vi "VisualizeModules.vi"() -> ()   [LabVIEW 2016]
uses:
  2_ModulePositioning/SingleModuleProgressReport.ctl
  <vilib>/vision/driver/NI_Vision_Acquisition_Software.lvlib
  <vilib>/vision/NI_Vision_Development_Module.lvlib
panel:
  in  "Calibration [um/pix]":dbl=0.25
  out "delta Y":sgl
  out "delta X":sgl
  out "Current Position":T1
  in  "Axis Speeds":T2={"X [mm/s]"=25.0, "Y [mm/s]"=12.5, "Z [mm/s]"=5.0}
  in  "stop":bool
  out "Placement Monitor":T3(plugin-control)
  out "appended path":path
  out "Fiducial Template":T3(plugin-control)
  in  "Templates path":path=path "C:/Users/Aerotech/Documents/BNL_ThermomechanicalStave/0_Calibration"
  in  "Module fiducial marker":T4(ring)=enum."[None]"
  out "Module Progress Report":T5(array[cluster])
  in  "Camera Name":refnum<k21>="cam0" caption="IMAQdx Session"
  in  "N modules":i32
  in  "Calibrated positions of fiducials [mm]":dbl[][](array[numeric])=[[-675.4228165149058, -196.82430550413875, -11.55], [-579.8428201474238, -196.8506568257386, -11.55], [-579.816468825824, -101.27066045825673, -11.55], [-675.3964651933059, -101.24430913665685, -11.55], [-577.422820239396, -196.8513240176017, -11.55], [-481.84282387191405, -196.87767533920157, -11.55], [-481.8164725503142, -101.29767897171968, -11.55], [-577.396468917796, -101.2713276501198, -11.55], [-479.42282396388623, -196.87834253106465, -11.55], [-383.8428275964043, -196.90469385266454, -11.55], [-383.81647627480436, -101.32469748518264, -11.55], [-479.3964726422863, -101.29834616358275, -11.55], [-381.42282768837646, -196.90536104452758, -11.55], [-285.8428313208945, -196.93171236612747, -11.55], [-285.8164799992946, -101.35171599864559, -11.55], [-381.39647636677654, -101.3253646770457, -11.55], [-283.4228314128667, -196.93237955799054, -11.55], [-187.84283504538473, -196.95873087959043, -11.55], [-187.8164837237848, -101.37873451210854, -11.55], [-283.39648009126677, -101.35238319050865, -11.55], [-185.42283513735697, -196.9593980714535, -11.55], [-89.84283876987502, -196.98574939305337, -11.55], [-89.81648744827521, -101.40575302557149, -11.55], [-185.39648381575705, -101.3794017039716, -11.55], [-87.42283886184703, -196.98641658491644, -11.55], [8.157157505634814, -197.01276790651633, -11.55], [8.183508827234618, -101.43277153903443, -11.55], [-87.39648754024722, -101.40642021743454, -11.55], [10.57715741366269, -197.01343509837938, -11.55], [106.15715378114453, -197.0397864199793, -11.55], [106.18350510274433, -101.45979005249738, -11.55], [10.603508735262494, -101.4334387308975, -11.55], [108.57715368917252, -197.04045361184234, -11.55], [204.15715005665436, -197.06680493344223, -11.55], [204.18350137825416, -101.48680856596033, -11.55], [108.60350501077232, -101.46045724436046, -11.55], [206.57714996468223, -197.0674721253053, -11.55], [302.1571463321641, -197.09382344690516, -11.55], [302.1834976537639, -101.5138270794233, -11.55], [206.60350128628204, -101.4874757578234, -11.55], [304.57714624019206, -197.09449063876826, -11.55], [400.1571426076739, -197.12084196036813, -11.55], [400.1834939292737, -101.54084559288623, -11.55], [304.60349756179187, -101.51449427128635, -11.55], [402.5771425157018, -197.1215091522312, -11.55], [498.15713888318373, -197.1478604738311, -11.55], [498.18349020478354, -101.56786410634919, -11.55], [402.6034938373016, -101.5415127847493, -11.55], [500.5771387912116, -197.14852766569413, -11.55], [596.1571351586933, -197.17487898729405, -11.55], [596.1834864802931, -101.59488261981214, -11.55], [500.6034901128114, -101.56853129821225, -11.55]]
  # "-101.244"
  # "-196.851"
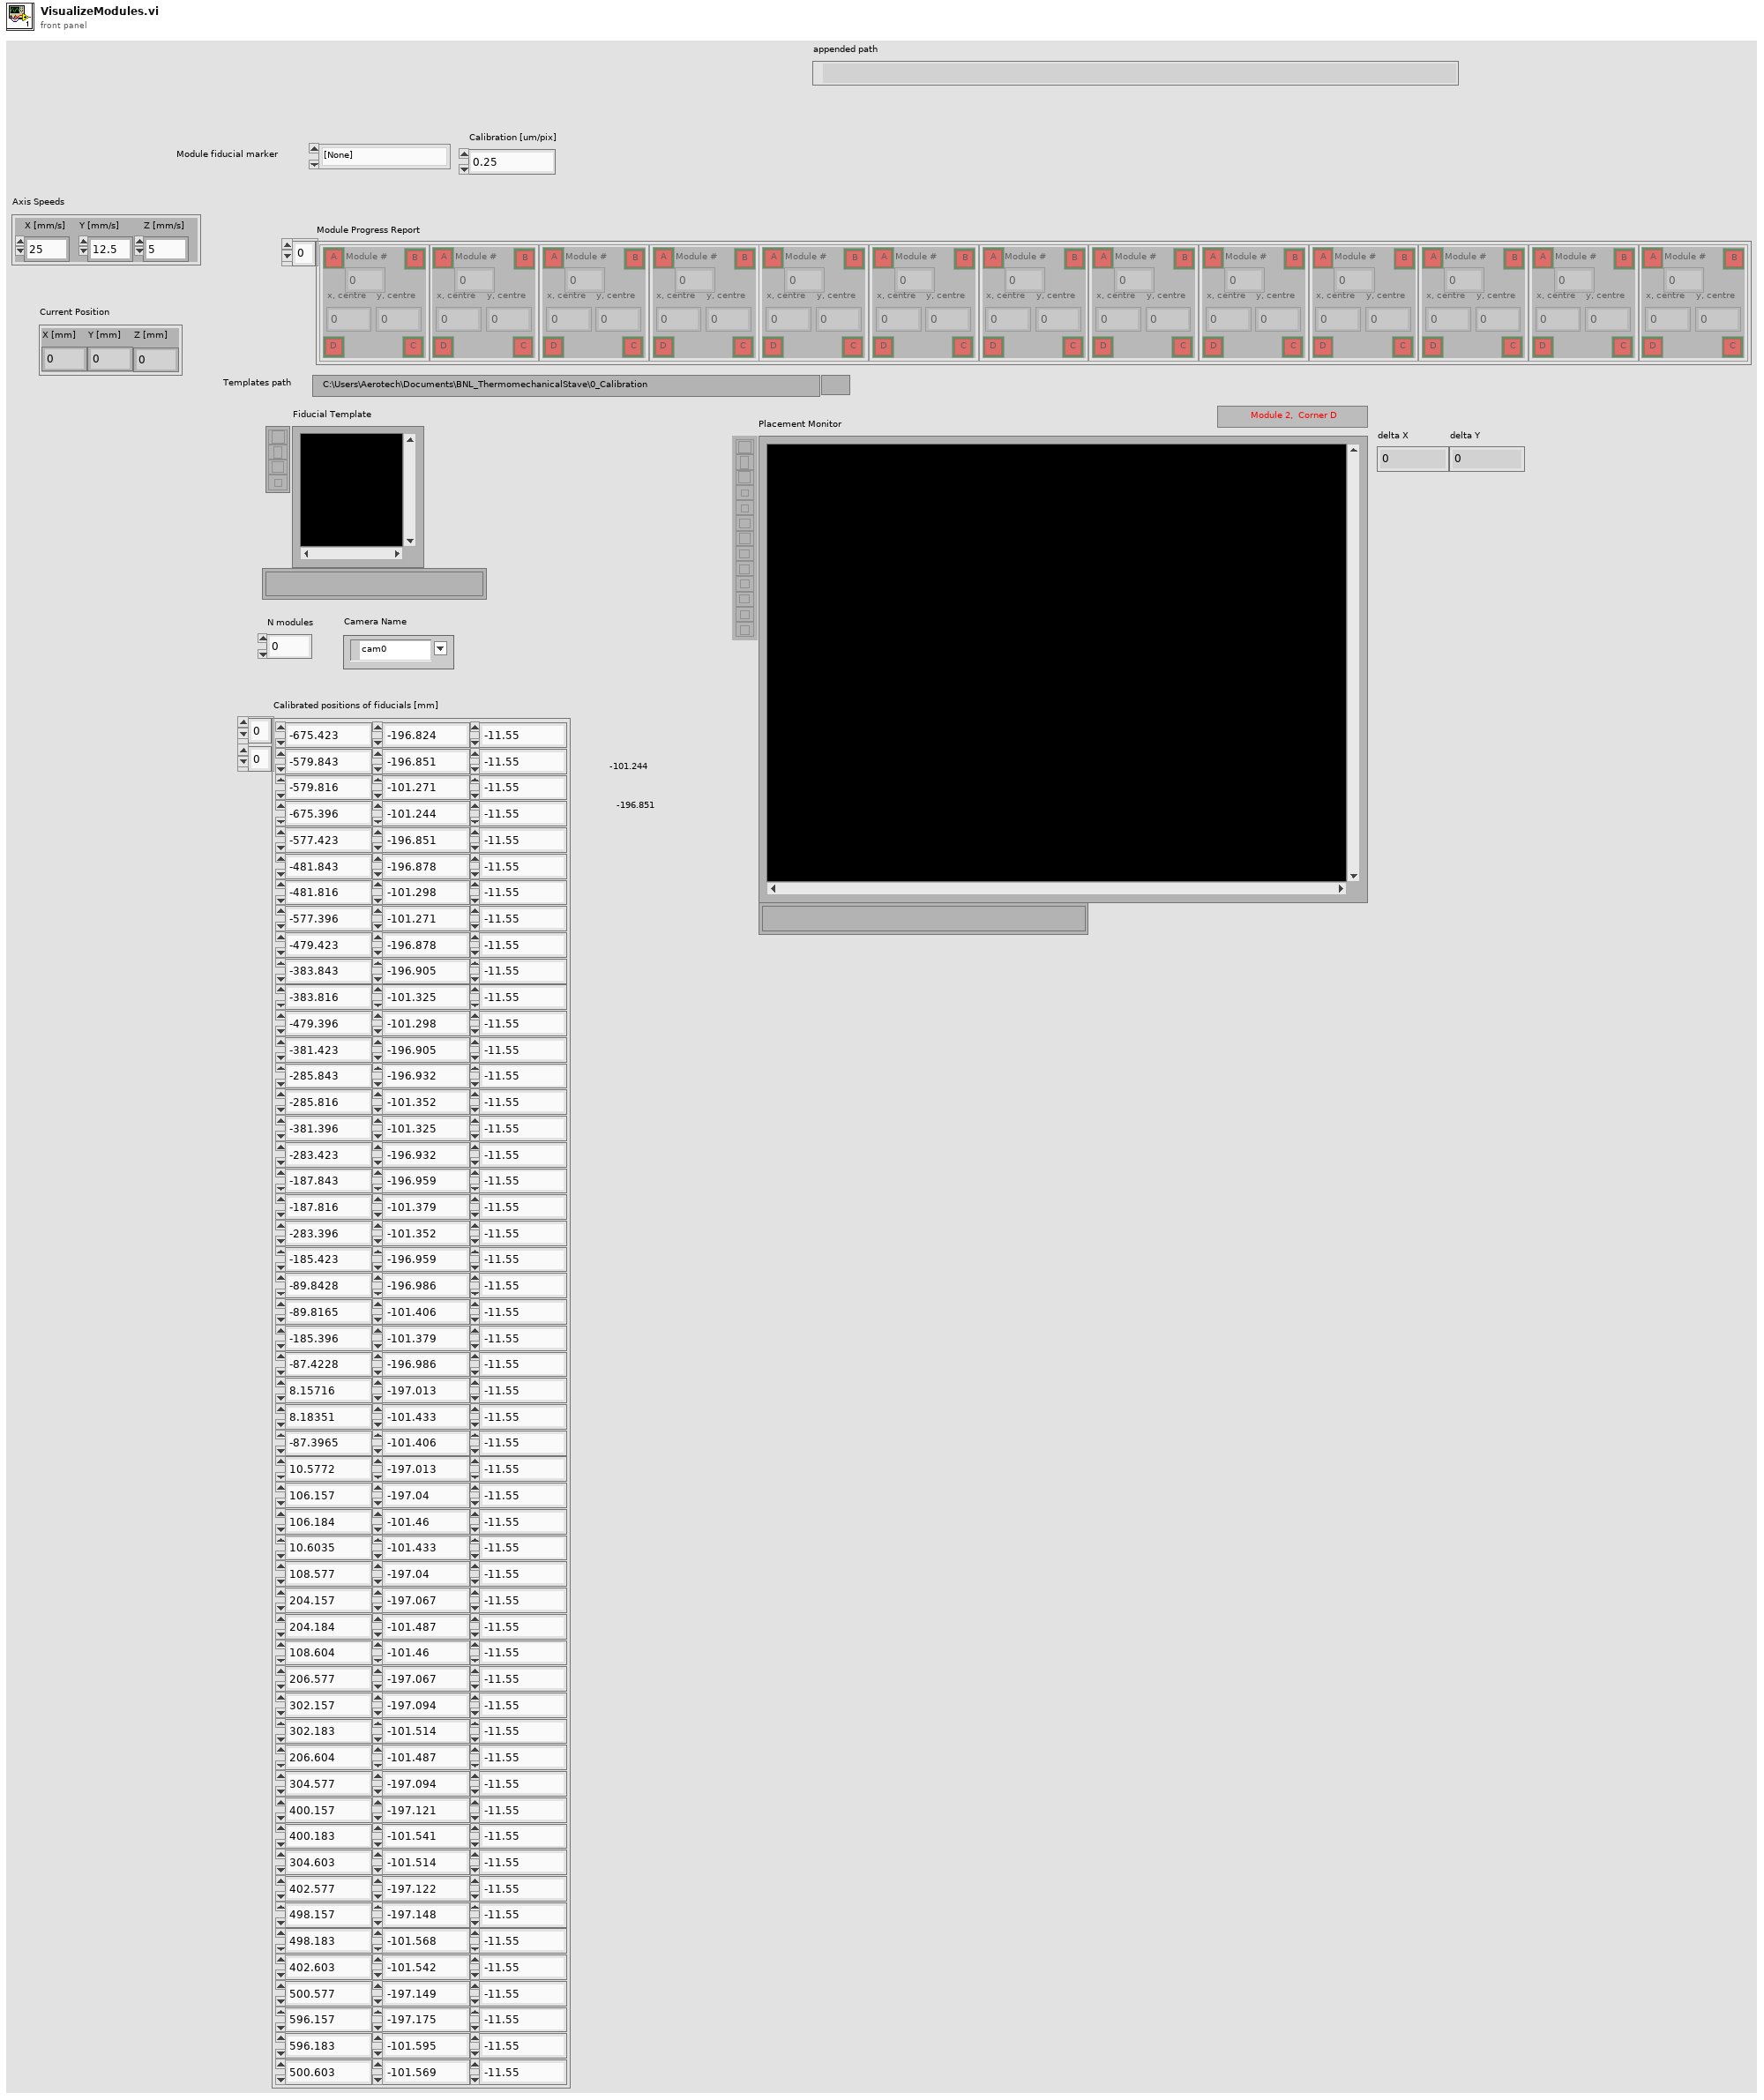
[diagram p1: front panel]
types:
  T1 = cluster{"X [mm]":dbl, "Y [mm]":dbl, "Z [mm]":dbl}
  T2 = cluster{"X [mm/s]":dbl, "Y [mm/s]":dbl, "Z [mm/s]":dbl}
  T3 = typedef "IMAQ Image.ctl" = refnum<image>
  T4 = enum16{"Mark C", "Mark B", "Strip Corner", "[None]"}
  T5 = cluster{"A":bool, "x, centre":dbl, "y, centre":dbl, "Module #":i32, "B":bool, "D":bool, "C":bool}[]
  T6 = typedef "SingleModuleProgressReport.ctl" = cluster{"A":bool, "x, centre":dbl, "y, centre":dbl, "Module #":i32, "B":bool, "D":bool, "C":bool}
  T7 = cluster{"Algorithm":i32, "Number of Matches Requested":i32, "Minimum Match Score":sgl, "SubPixel Accuracy":bool, "Rotation Angle Ranges":cluster{"Start":sgl, "End":sgl}[], "Show Search Area":bool, "Show Result":bool}
  T8 = typedef "IMAQdx.ctl" = refnum<k21>
  T9 = cluster{"Final X":dbl, "Final Y":dbl, "Final Z":dbl}
  T10 = cluster{"Position":cluster{"x":sgl, "y":sgl}, "Angle":sgl, "Scale":sgl, "Score":sgl, "Bounding Box":cluster{"x":sgl, "y":sgl}[]}[]
  T11 = cluster{"Position":cluster{"x":sgl, "y":sgl}, "Angle":sgl, "Scale":sgl, "Score":sgl, "Bounding Box":cluster{"x":sgl, "y":sgl}[]}
  T12 = cluster{"A":bool, "x, centre":dbl, "y, centre":dbl, "Module #":i32, "B":bool, "D":bool, "C":bool}
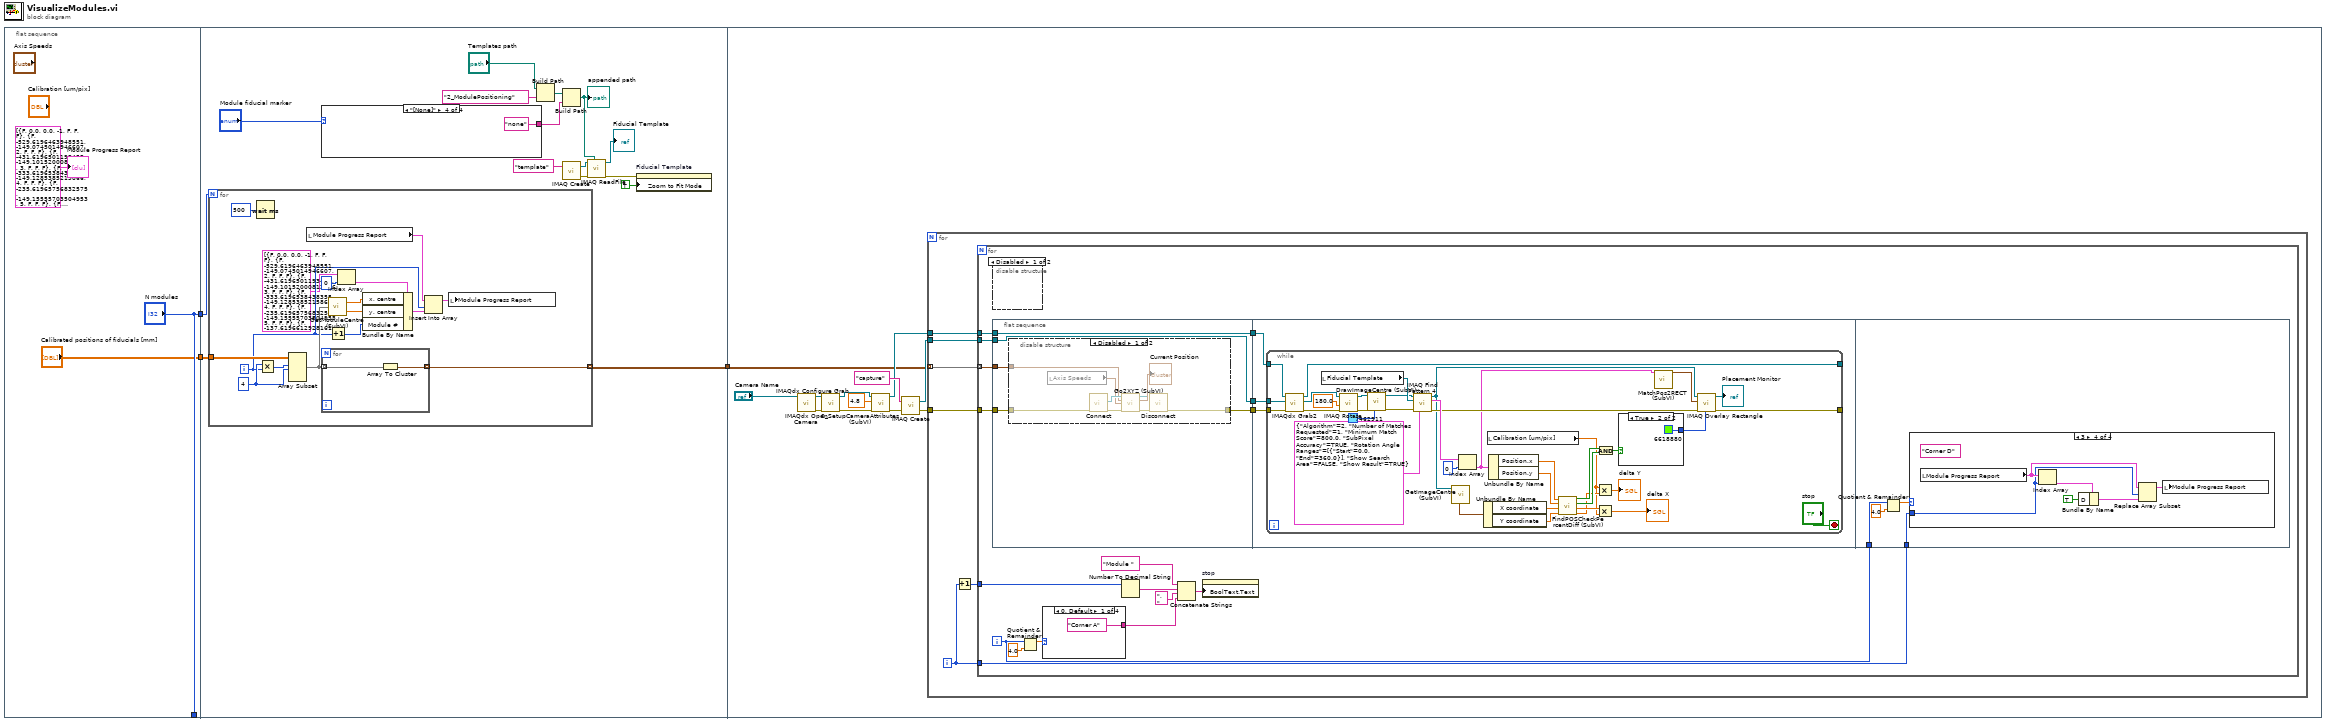
[diagram p0: block diagram]
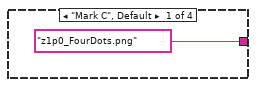
[diagram p2: hidden frame]
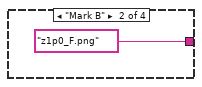
[diagram p3: hidden frame]
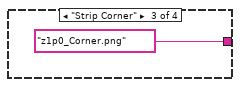
[diagram p4: hidden frame]
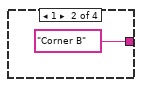
[diagram p6: hidden frame]
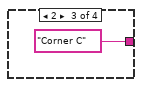
[diagram p7: hidden frame]
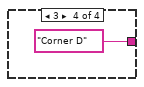
[diagram p8: hidden frame]
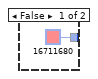
[diagram p10: hidden frame]
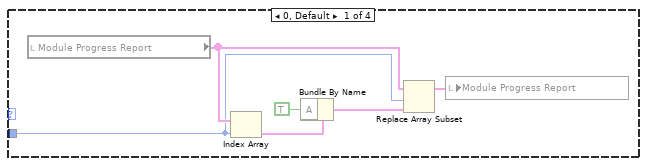
[diagram p11: hidden frame]
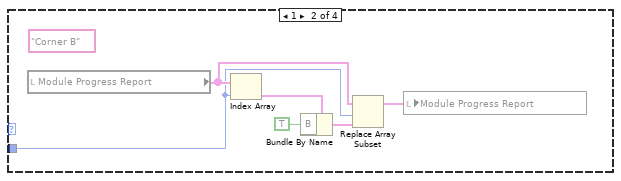
[diagram p12: hidden frame]
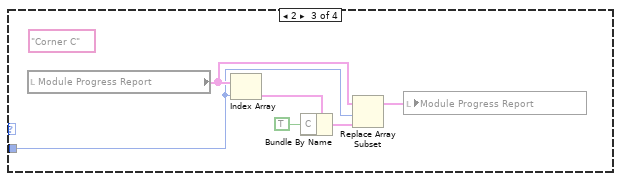
[diagram p13: hidden frame]
diagram:
  n1 = flat-sequence {
    tunnel: ["N modules"] -> _
    tunnel: ["N modules"] -> w2
    tunnel: ["Calibrated positions of fiducials [mm]"] -> w1
    tunnel: [w19] -> w3
    tunnel: w2 -> [w21]
    tunnel: w1 -> [w20]
    tunnel: w3 -> [w44]
    frame #0 {
      "Module Progress Report" <- T6[] [{"A"=FALSE, "x, centre"=0.0, "y, centre"=0.0, "Module #"=-1, "B"=FALSE, "D"=FALSE, "C"=FALSE}, {"A"=FALSE, "x, centre"=-529.6196463948551, "y, centre"=-149.0745014946607, "Module #"=2, "B"=FALSE, "D"=FALSE, "C"=FALSE}, {"A"=FALSE, "x, centre"=-431.6196501193453, "y, centre"=-149.10152000812366, "Module #"=3, "B"=FALSE, "D"=FALSE, "C"=FALSE}, {"A"=FALSE, "x, centre"=-333.6196538438355, "y, centre"=-149.1285385215866, "Module #"=4, "B"=FALSE, "D"=FALSE, "C"=FALSE}, {"A"=FALSE, "x, centre"=-235.61965756832575, "y, centre"=-149.15555703504953, "Module #"=5, "B"=FALSE, "D"=FALSE, "C"=FALSE}, {"A"=FALSE, "x, centre"=-137.6196612928161, "y, centre"=-149.1825755485125, "Module #"=6, "B"=FALSE, "D"=FALSE, "C"=FALSE}, {"A"=FALSE, "x, centre"=-627.6196426703649, "y, centre"=-149.04748298119773, "Module #"=1, "B"=FALSE, "D"=FALSE, "C"=FALSE}, {"A"=FALSE, "x, centre"=-529.6196463948551, "y, centre"=-149.0745014946607, "Module #"=2, "B"=FALSE, "D"=FALSE, "C"=FALSE}, {"A"=FALSE, "x, centre"=-431.6196501193453, "y, centre"=-149.10152000812366, "Module #"=3, "B"=FALSE, "D"=FALSE, "C"=FALSE}, {"A"=FALSE, "x, centre"=-333.6196538438355, "y, centre"=-149.1285385215866, "Module #"=4, "B"=FALSE, "D"=FALSE, "C"=FALSE}, {"A"=FALSE, "x, centre"=-235.61965756832575, "y, centre"=-149.15555703504953, "Module #"=5, "B"=FALSE, "D"=FALSE, "C"=FALSE}, {"A"=FALSE, "x, centre"=-137.6196612928161, "y, centre"=-149.1825755485125, "Module #"=6, "B"=FALSE, "D"=FALSE, "C"=FALSE}, {"A"=FALSE, "x, centre"=-39.619665017306204, "y, centre"=-149.20959406197545, "Module #"=7, "B"=FALSE, "D"=FALSE, "C"=FALSE}, {"A"=FALSE, "x, centre"=58.38033125820351, "y, centre"=-149.2366125754384, "Module #"=8, "B"=FALSE, "D"=FALSE, "C"=FALSE}, {"A"=FALSE, "x, centre"=156.38032753371334, "y, centre"=-149.26363108890132, "Module #"=9, "B"=FALSE, "D"=FALSE, "C"=FALSE}, {"A"=FALSE, "x, centre"=254.38032380922306, "y, centre"=-149.29064960236428, "Module #"=10, "B"=FALSE, "D"=FALSE, "C"=FALSE}, {"A"=FALSE, "x, centre"=352.3803200847329, "y, centre"=-149.31766811582725, "Module #"=11, "B"=FALSE, "D"=FALSE, "C"=FALSE}, {"A"=FALSE, "x, centre"=450.38031636024266, "y, centre"=-149.3446866292902, "Module #"=12, "B"=FALSE, "D"=FALSE, "C"=FALSE}, {"A"=FALSE, "x, centre"=548.3803126357524, "y, centre"=-149.37170514275314, "Module #"=13, "B"=FALSE, "D"=FALSE, "C"=FALSE}] ("Module Progress Report")
    }
    frame #1 {
      n2 = for {
        N: w21 -> [_]
        tunnel: w20 -> [w41]
        tunnel: [w38] -> w19 mode=indexing
        i -> [w29]
        w39 = 4 ("x")
        n3 = Wait (ms)(milliseconds to wait=u32 500) -> ()  [unwired: 1 out]
        n4 = Multiply(x=w39, y=w29) -> (x*y=w40:i32)
        n5 = Array Subset(array=w41, index (row)=w40, length (row)=w39) -> (w37:dbl[][])  [unwired: 2 in]
        n6 = local read "Module Progress Report"() -> (w30:T5)
        n7 = for {
          tunnel: w37 -> [w42] mode=indexing
          tunnel: [w43] -> w38 mode=indexing
          n8 = Array To Cluster(array=w42) -> (cluster=w43:cluster{"[0]":dbl, "[1]":dbl, "[2]":dbl})
        }
        n9 = call "GetModuleCentre (SubVI).vi"("4x3 Array of Fiducial Coordinates"=w37) -> ("x, centre"=w36:dbl, "y, centre"=w35:dbl)
        n10 = Increment(x=w29) -> (x+1=w34:i32)
        n11 = Index Array(array=T6[] [{"A"=FALSE, "x, centre"=0.0, "y, centre"=0.0, "Module #"=-1, "B"=FALSE, "D"=FALSE, "C"=FALSE}, {"A"=FALSE, "x, centre"=-529.6196463948551, "y, centre"=-149.0745014946607, "Module #"=2, "B"=FALSE, "D"=FALSE, "C"=FALSE}, {"A"=FALSE, "x, centre"=-431.6196501193453, "y, centre"=-149.10152000812366, "Module #"=3, "B"=FALSE, "D"=FALSE, "C"=FALSE}, {"A"=FALSE, "x, centre"=-333.6196538438355, "y, centre"=-149.1285385215866, "Module #"=4, "B"=FALSE, "D"=FALSE, "C"=FALSE}, {"A"=FALSE, "x, centre"=-235.61965756832575, "y, centre"=-149.15555703504953, "Module #"=5, "B"=FALSE, "D"=FALSE, "C"=FALSE}, {"A"=FALSE, "x, centre"=-137.6196612928161, "y, centre"=-149.1825755485125, "Module #"=6, "B"=FALSE, "D"=FALSE, "C"=FALSE}, {"A"=FALSE, "x, centre"=-627.6196426703649, "y, centre"=-149.04748298119773, "Module #"=1, "B"=FALSE, "D"=FALSE, "C"=FALSE}, {"A"=FALSE, "x, centre"=-529.6196463948551, "y, centre"=-149.0745014946607, "Module #"=2, "B"=FALSE, "D"=FALSE, "C"=FALSE}, {"A"=FALSE, "x, centre"=-431.6196501193453, "y, centre"=-149.10152000812366, "Module #"=3, "B"=FALSE, "D"=FALSE, "C"=FALSE}, {"A"=FALSE, "x, centre"=-333.6196538438355, "y, centre"=-149.1285385215866, "Module #"=4, "B"=FALSE, "D"=FALSE, "C"=FALSE}, {"A"=FALSE, "x, centre"=-235.61965756832575, "y, centre"=-149.15555703504953, "Module #"=5, "B"=FALSE, "D"=FALSE, "C"=FALSE}, {"A"=FALSE, "x, centre"=-137.6196612928161, "y, centre"=-149.1825755485125, "Module #"=6, "B"=FALSE, "D"=FALSE, "C"=FALSE}, {"A"=FALSE, "x, centre"=-39.619665017306204, "y, centre"=-149.20959406197545, "Module #"=7, "B"=FALSE, "D"=FALSE, "C"=FALSE}, {"A"=FALSE, "x, centre"=58.38033125820351, "y, centre"=-149.2366125754384, "Module #"=8, "B"=FALSE, "D"=FALSE, "C"=FALSE}, {"A"=FALSE, "x, centre"=156.38032753371334, "y, centre"=-149.26363108890132, "Module #"=9, "B"=FALSE, "D"=FALSE, "C"=FALSE}, {"A"=FALSE, "x, centre"=254.38032380922306, "y, centre"=-149.29064960236428, "Module #"=10, "B"=FALSE, "D"=FALSE, "C"=FALSE}, {"A"=FALSE, "x, centre"=352.3803200847329, "y, centre"=-149.31766811582725, "Module #"=11, "B"=FALSE, "D"=FALSE, "C"=FALSE}, {"A"=FALSE, "x, centre"=450.38031636024266, "y, centre"=-149.3446866292902, "Module #"=12, "B"=FALSE, "D"=FALSE, "C"=FALSE}, {"A"=FALSE, "x, centre"=548.3803126357524, "y, centre"=-149.37170514275314, "Module #"=13, "B"=FALSE, "D"=FALSE, "C"=FALSE}] ("Module Progress Report"), index=0) -> (element=w31:T6)
        n12 = Bundle By Name(cluster=w31, "x, centre"=w36, "y, centre"=w35, "Module #"=w34) -> (w26:T6)
        n13 = Insert Into Array(array=w30, index=w29, new element=w26) -> (w28:T5)
        n14 = local write "Module Progress Report"(w28) -> ()
      }
      n15 = case shown="\"[None]\"" "Module fiducial marker" {
        tunnel: ["z1p0_FourDots.png" ("name or relative path") "z1p0_F.png" ("name or relative path") "z1p0_Corner.png" ("name or relative path") "none" ("name or relative path")] -> w18
        frame "Mark C", Default {
        }
        frame "Mark B" {
        }
        frame "Strip Corner" {
        }
        frame "[None]" {
        }
      }
      n16 = Build Path(base path="Templates path", name or relative path="2_ModulePositioning") -> (appended path=w16:path)
      n17 = Build Path(base path=w16, name or relative path=w18) -> (appended path=w14:path)
      "appended path" <- w14
      n18 = call "IMAQ Create"("Image Name"="template") -> ("New Image"=w13:T3, "error out"=w12:errorcluster)  [unwired: 4 in]
      n19 = call "IMAQ ReadFile"("File Path"=w14, "error in (no error)"=w12, "Image"=w13) -> ("error out"=w8:errorcluster, "Image Out"=→"Fiducial Template":T3)  [unwired: 4 in, 3 out]
      n20 = property on="Fiducial Template" class="ImageControl"(error in=w8, "Zoom to Fit Mode"=TRUE) -> ()  [unwired: 1 in, 2 out]
    }
    frame #2 {
      n21 = call <vilib>:"IMAQdx Open Camera.vi"("Session In"="Camera Name") -> ("error out"=w53:errorcluster, "Session Out"=w54:T8)  [unwired: 2 in, 7 out]
      n22 = call <vilib>:"IMAQdx Configure Grab.vi"("error in"=w53, "Session In"=w54) -> ("error out"=w51:errorcluster, "Session Out"=w52:T8)  [unwired: 8 out]
      n23 = call "0_SetupCameraAttributes (SubVI).vi"("error in (no error)"=w51, "Gain"=4.8, "Camera session in"=w52) -> ("error out"=w49:errorcluster, "Camera session out"=w46:T8)  [unwired: 7 in]
      n24 = call "IMAQ Create"("Image Name"="capture", "error in (no error)"=w49) -> ("New Image"=w47:T3, "error out"=w45:errorcluster)  [unwired: 3 in]
      n25 = for {
        tunnel: w46 -> [w61]
        tunnel: w47 -> [w60]
        tunnel: w45 -> [w59]
        tunnel: w44 -> [w57] mode=indexing
        i -> [w56]
        n26 = Increment(x=w56) -> (x+1=w58:i32)
        n27 = for {
          tunnel: w61 -> [w75]
          tunnel: w60 -> [w74]
          tunnel: w59 -> [w73]
          tunnel: w58 -> [w68]
          tunnel: w57 -> [w64] mode=indexing
          tunnel: w56 -> [w63]
          i -> [w62]
          n28 = disable-structure shown="Disabled" {
            frame Disabled {
            }
            frame Enabled {
            }
          }
          n29 = flat-sequence {
            tunnel: w75 -> [w86]
            tunnel: w73 -> [w85]
            tunnel: w74 -> [w87]
            tunnel: [w87] -> w78
            tunnel: [w84] -> w77
            tunnel: [w86] -> w76
            tunnel: w64 -> [w83]
            tunnel: w78 -> [w100]
            tunnel: w77 -> [w99]
            tunnel: w76 -> [w98]
            tunnel: w63 -> [w141]
            tunnel: w62 -> [w140]
            frame #0 {
              n30 = disable-structure shown="Disabled" {
                disable-tunnel: w85 -> [w96 w97]
                disable-tunnel: [w95 w97] -> w84
                disable-tunnel: w83 -> [w89 _]
                frame Disabled {
                  n31 = local read "Axis Speeds"() -> (w88:T2)
                  n32 = call "Connect.vi"("error in (no error)"=w96) -> ("error out"=w93:errorcluster, "controller"=w92:refnum<k24>)  [unwired: 9 in]
                  n33 = call "Go2XYZ (SubVI).vi"(".NET Refnum in"=w92, "Go to Coordinates"=w89, "Axis Speeds"=w88, "error in (no error)"=w93) -> (".NET Refnum out"=w91:refnum<k24>, "Final Position"=→"Current Position":T9, "error out"=w90:errorcluster)  [unwired: 7 in, 2 out]
                  n34 = call "Disconnect.vi"("error in (no error)"=w90, "controller"=w91) -> ("error out"=w95:errorcluster)  [unwired: 9 in]
                }
                frame Enabled {
                }
              }
            }
            frame #1 {
              n35 = while {
                tunnel: w100 -> [w137]
                tunnel: w99 -> [w136]
                tunnel: w98 -> [w135]
                tunnel: [w131] -> _
                tunnel: [w123] -> _
                stop <- "stop" stop-if-true
                n36 = call <vilib>:"IMAQdx Grab2.vi"("error in"=w136, "Image In"=w137, "Session In"=w135) -> ("error out"=w132:errorcluster, "Image Out"=w134:T3, "Session Out"=w131:T8)  [unwired: 5 in, 1 out]
                n37 = local read "Fiducial Template"() -> (w128:T3)
                n38 = call "IMAQ Rotate"("error in (no error)"=w132, "Angle (degrees)"=sgl 180.0, "Image Src"=w134) -> ("error out"=w103:errorcluster, "Image Dst Out"=w105:T3)  [unwired: 7 in]
                n39 = call "DrawImageCentre (SubVI).vi"("Axis colour"=u32 7462911, "error in (no error)"=w103, "Refnum in"=w105) -> ("error out"=w102:errorcluster, "Refnum out"=w104:T3)  [unwired: 7 in]
                n40 = call "IMAQ Find Pattern 4"("Image"=w104, "Template"=w128, "error in"=w102, "Settings"=T7 {"Algorithm"=2, "Number of Matches Requested"=1, "Minimum Match Score"=800.0, "SubPixel Accuracy"=TRUE, "Rotation Angle Ranges"=[{"Start"=0.0, "End"=360.0}], "Show Search Area"=FALSE, "Show Result"=TRUE}) -> ("Image Out"=w117:T3, "Matches (pixel)"=w126:T10, "error out"=w124:errorcluster)  [unwired: 5 in, 4 out]
                n41 = call "GetImageCentre (SubVI).vi"("Image in \n(refnum)"=w117) -> ("Centre Point"=w116:cluster{"X coordinate":dbl, "Y coordinate":dbl})  [unwired: 4 in, 4 out]
                n42 = Index Array(array=w126, index=0) -> (element=w111:T11)
                n43 = Unbundle By Name(w116) -> ("X coordinate"=w115:dbl, "Y coordinate"=w114:dbl)
                n44 = local read "Calibration [um/pix]"() -> (w108:dbl)
                n45 = Unbundle By Name(w111) -> ("Position.x"=w121:sgl, "Position.y"=w120:sgl)
                n46 = call "FindPOSCheckPercentDiff (SubVI).vi"("x"=w121, "y"=w120, "true x"=w115, "true y"=w114) -> ("pass x coordinate"=w119:bool, "pass y coordinate"=w118:bool, "delta X"=w110:sgl, "delta Y"=w109:sgl)  [unwired: 3 in]
                n47 = Multiply(x=w108, y=w109) -> (x*y=→"delta Y":dbl)
                n48 = Multiply(x=w110, y=w108) -> (x*y=→"delta X":dbl)
                n49 = And(x=w119, y=w118) -> (x .and. y?=w113:bool)
                n50 = case shown="True" w113 {
                  tunnel: [u32 16711680 ("Color") u32 6618880 ("Color")] -> w112
                  frame False {
                  }
                  frame True {
                  }
                }
                n51 = call "MatchPos2RECT (SubVI).vi"("Match element"=w111) -> ("Rectangle"=w127:cluster{"x":sgl, "y":sgl, dbl, dbl})  [unwired: 10 in]
                n52 = call "IMAQ Overlay Rectangle"("Color"=w112, "error in (no error)"=w124, "Rectangle"=w127, "Image"=w117) -> ("error out"=w123:errorcluster, "Image Out"=→"Placement Monitor":T3)  [unwired: 6 in]
              }
            }
            frame #2 {
              n53 = Quotient & Remainder(x=w140, y=4.0) -> (x-y*floor(x/y)=w143:dbl)  [unwired: 1 out]
              n54 = case shown="3" w143 {
                tunnel: w141 -> [w146 w150 w156 w162]
                frame 0, Default {
                  n55 = local read "Module Progress Report"() -> (w147:T5)
                  n56 = Index Array(array=w147, index=w146) -> (element=w145:T12)
                  n57 = Bundle By Name(cluster=w145, "A"=TRUE) -> (w148:T12)
                  n58 = Replace Array Subset(array=w147, new element=w148, index=w146) -> (w144:T5)
                  n59 = local write "Module Progress Report"(w144) -> ()
                }
                frame 1 {
                  (unwired) "Corner B"
                  n60 = local read "Module Progress Report"() -> (w153:T5)
                  n61 = Index Array(array=w153, index=w150) -> (element=w152:T12)
                  n62 = Bundle By Name(cluster=w152, "B"=TRUE ("A")) -> (w154:T12)
                  n63 = Replace Array Subset(array=w153, new element=w154, index=w150) -> (w151:T5)
                  n64 = local write "Module Progress Report"(w151) -> ()
                }
                frame 2 {
                  (unwired) "Corner C"
                  n65 = local read "Module Progress Report"() -> (w159:T5)
                  n66 = Index Array(array=w159, index=w156) -> (element=w158:T12)
                  n67 = Bundle By Name(cluster=w158, "C"=TRUE ("A")) -> (w160:T12)
                  n68 = Replace Array Subset(array=w159, new element=w160, index=w156) -> (w157:T5)
                  n69 = local write "Module Progress Report"(w157) -> ()
                }
                frame 3 {
                  (unwired) "Corner D"
                  n70 = local read "Module Progress Report"() -> (w165:T5)
                  n71 = Index Array(array=w165, index=w162) -> (element=w164:T12)
                  n72 = Bundle By Name(cluster=w164, "D"=TRUE ("A")) -> (w166:T12)
                  n73 = Replace Array Subset(array=w165, new element=w166, index=w162) -> (w163:T5)
                  n74 = local write "Module Progress Report"(w163) -> ()
                }
              }
            }
          }
          n75 = Quotient & Remainder(x=w62, y=4.0) -> (x-y*floor(x/y)=w65:dbl)  [unwired: 1 out]
          n76 = case shown="0, Default" w65 {
            tunnel: ["Corner A" "Corner B" "Corner C" "Corner D"] -> w67
            frame 0, Default {
            }
            frame 1 {
            }
            frame 2 {
            }
            frame 3 {
            }
          }
          n77 = Number To Decimal String(number=w68) -> (decimal integer string=w71:string)  [unwired: 1 in]
          n78 = Concatenate Strings("Module " ("string"), w71, ",  " ("string"), w67) -> (w72:string)
          n79 = property on="stop" class="Bool"("BoolText.Text"=w72) -> ()  [unwired: 2 in, 2 out]
        }
      }
    }
  }
